vi "dfd_Change Phase View.vi"(10 "phase view":T1, 11 "phase in (rad)":dbl[](array[numeric]) format="%.2f") -> (3 "phase out":dbl[](array[numeric]) format="%.2f")   [LabVIEW 2017, in "NI_DigFilterLicensed.lvlib"]
uses:
  <vilib>/addons/Digital Filter Design/NI_DigFilterLicensed.lvlib
  <vilib>/addons/Digital Filter Design/_Objects.llb/DFD Phase Setting.ctl
  <vilib>/Analysis/NI_AALPro.lvlib
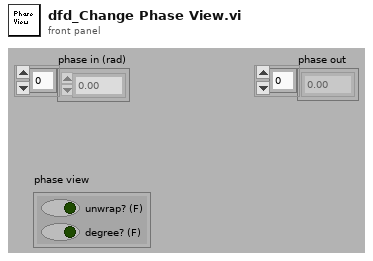
[diagram p1: front panel]
types:
  T1 = typedef "NI_DigFilterLicensed.lvlib/DFD Phase Setting.ctl" = cluster{"unwrap? (F)":bool, "degree? (F)":bool}
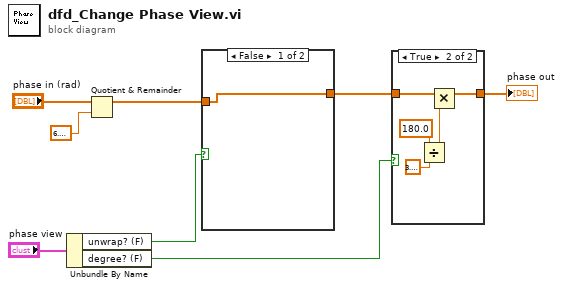
[diagram p0: block diagram]
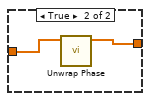
[diagram p2: hidden frame]
diagram:
  n1 = Unbundle By Name("phase view") -> ("unwrap? (F)"=w5:bool, "degree? (F)"=w1:bool)
  n2 = Quotient & Remainder(x="phase in (rad)", y=6.283185307179586) -> (x-y*floor(x/y)=w4:dbl[])  [unwired: 1 out]
  n3 = case shown="False" w5 {
    tunnel: w4 -> [w9 w11]
    tunnel: [w9 w10] -> w3
    frame False {
    }
    frame True {
      n4 = call <vilib>:"Unwrap Phase.vi"("Phase"=w11) -> ("Unwrapped Phase"=w10:dbl[])  [unwired: 1 in, 9 out]
    }
  }
  n5 = case shown="True" w1 {
    tunnel: w3 -> [w12 w16]
    tunnel: [w12 w17] -> w2
    frame False {
    }
    frame True {
      n6 = Divide(x=180.0, y=3.141592653589793 ("end")) -> (x/y=w13:dbl)
      n7 = Multiply(x=w16, y=w13) -> (x*y=w17:dbl[])
    }
  }
  "phase out" <- w2
